vi "Download Web Data V.vi"(0 "minute":i32, 1 "year":i32, 2 "password":string, 5 "hour":i32, 7 "day":i32, 9 "month":i32, 11 "error in (no error)":errorcluster, 12 "userName":string) -> (4 "password out":string, 6 "function return":i32, 14 "userName out":string, 15 "error out":errorcluster)   [LabVIEW 2009, in "VantagePro.lvlib"]
doc: "DllAccess int _stdcall DownloadWebData_V(DateTimeStamp dateTimeStamp, char *userName, char *password);"
uses:
  VantagePro.lvlib
  <userlib>/VantagePro/VantagePro.dll
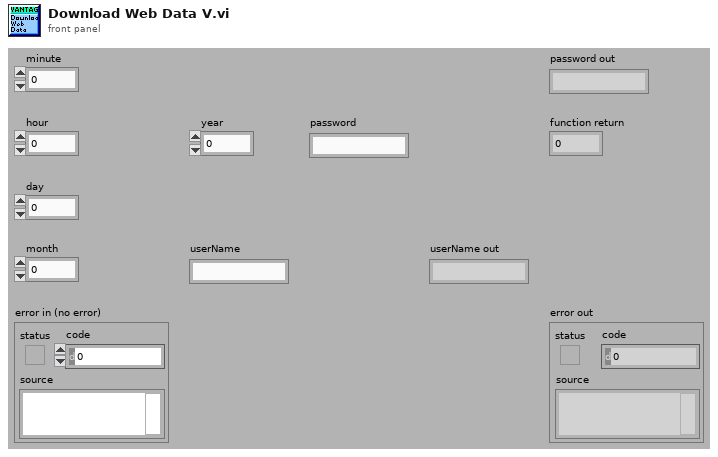
[diagram p1: front panel]
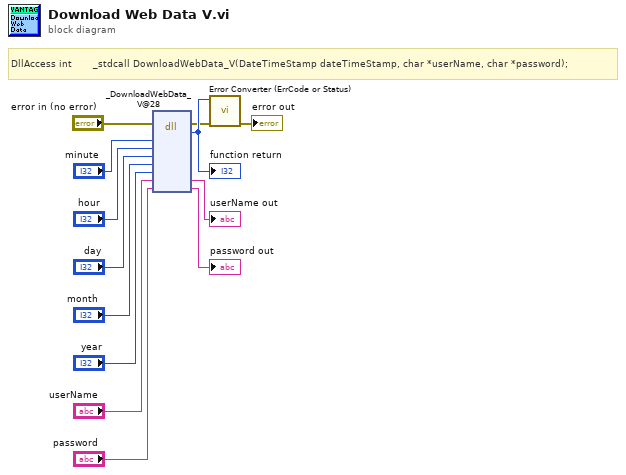
[diagram p0: block diagram]
diagram:
  # "DllAccess int       _stdcall DownloadWebData_V(DateTimeStamp dateTimeStamp, char *userName, char *password);"
  n1 = dll-call lib="C:/Program Files/National Instruments/LabVIEW 2010/user.lib/VantagePro/VantagePro.*" fn="_DownloadWebData_V@28"(error in="error in (no error)", "minute"="minute", "hour"="hour", "day"="day", "month"="month", "year"="year", "userName"="userName", "password"="password") -> (error out=w2:errorcluster, w13:i32, "userName"=→"userName out":string, "password"=→"password out":string)  [unwired: 7 in, 1 out]
  "function return" <- w13
  n2 = call "Error Converter (ErrCode or Status).vi"("error in (no error)"=w2, "error code"=w13) -> ("error out"=→"error out":errorcluster)  [unwired: 9 in]
